vi "ecg.vi"() -> ()   [LabVIEW 2023]
uses:
  <vilib>/Analysis/3filter.llb/Filter Passband Type.ctl
  <vilib>/Utility/file.llb/Read Delimited Spreadsheet (DBL).vi
  <vilib>/Analysis/3filter.llb/Butterworth Filter (DBL).vi
  <vilib>/Analysis/NI_AALBase.lvlib
  <vilib>/Analysis/NI_AAL_SigProc.lvlib
panel:
  out "HR":dbl
  out "Hz":dbl
  in  "filter type":T1
  in  "low cutoff freq: fl":dbl=0.12500000000000006 format="%0.4f"
  in  "high cutoff freq: fh":dbl=0.45000000000000007 format="%0.2f"
  in  "sampling freq: fs":dbl=1.0 format="%0.2f"
  out "Visualization":dbl[][](graph)
  in  "Path":path
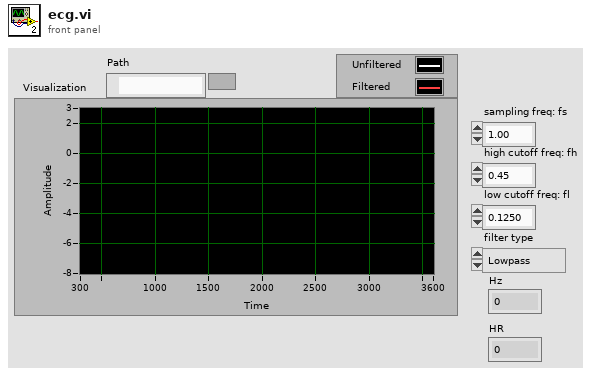
[diagram p1: front panel]
types:
  T1 = typedef "NI_AALBase.lvlib/Filter Passband Type.ctl" = enum32{"Lowpass", "Highpass", "Bandpass", "Bandstop"}
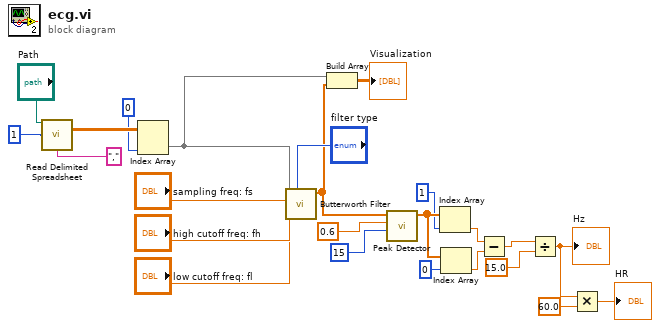
[diagram p0: block diagram]
diagram:
  n1 = call-poly <vilib>:"Read Delimited Spreadsheet.vi"("file path (dialog if empty)"="Path", "start of read offset (chars.:0)"=1, "delimiter (\\t)"="," ("delimiter (\\t)")) -> ("all rows"=w21:dbl[][])  [unwired: 7 in, 5 out]
  n2 = Index Array(array=w21, index (col)=0) -> (element=w15:dbl[])  [unwired: 1 in]
  n3 = call-poly <vilib>:"Butterworth Filter.vi"("filter type"="filter type", "low cutoff freq: fl"="low cutoff freq: fl", "high cutoff freq: fh"="high cutoff freq: fh", "sampling freq: fs"="sampling freq: fs", "X"=w15) -> ("Filtered X"=w13:dbl[])  [unwired: 3 in, 1 out]
  n4 = Build Array(w15, w13) -> (→"Visualization":dbl[][])
  n5 = call <vilib>:"Peak Detector.vi"("width"=15, "threshold"=0.6, "X"=w13) -> ("Locations"=w10:dbl[])  [unwired: 4 in, 4 out]
  n6 = Index Array(array=w10, index=1) -> (element=w7:dbl)
  n7 = Index Array(array=w10, index=0) -> (element=w6:dbl)
  n8 = Subtract(x=w7, y=w6) -> (x-y=w5:dbl)
  n9 = Divide(x=w5, y=15.0) -> (x/y=w3:dbl)
  "Hz" <- w3
  n10 = Multiply(x=w3, y=60.0) -> (x*y=→"HR":dbl)
